vi "AG33XXX.enable output.vi"(0 "i ref in":refnum<vi>, 2 "outputEnable":bool, 3 "ms timeout (10000)":i32=10000, 5 "error in (no error)":errorcluster) -> (14 "i ref out":refnum<vi>, 17 "timed out":bool, 19 "error out":errorcluster)   [LabVIEW 2014, in "AG33XXX.lvlib"]
doc: "Enables the output of the device."
uses:
  AG33XXX.lvlib
  CS_Core/CSApplicationBaseClasses/AFGBase/AFGBase.serviceType.ctl
  CS_Core/CSApplicationBaseClasses/AFGBase/AFGBase.directionType.ctl
  CSlibraries/UtilityLib/UtilityLib.valueStatus.ctl
  CS_Core/CSApplicationBaseClasses/DeviceBase/DeviceBase.lvlib
  CS_Core/CSApplicationBaseClasses/AFGBase/AFGBase.lvlib
  CSlibraries/UtilityLib/UtilityLib.lvlib
  instr.lib/agilent_33xxx_series/Agilent 33XXX Series/Agilent 33XXX Series.lvlib
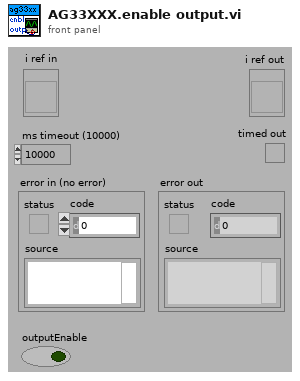
[diagram p1: front panel]
types:
  T1 = typedef "UtilityLib.lvlib/UtilityLib.valueStatus.ctl" = enum16{"no info available", "stand by/off", "on", "warning", "alarm/malfunction", "not implemented", "user action required", "important information", "system default", "control default", "indicator default", "button default"}
  T2 = typedef "AFGBase.lvlib/AFGBase.directionType.ctl" = enum16{"unknown", "update actual value", "update nominal value", "update both"}
  T3 = typedef "AFGBase.lvlib/AFGBase.serviceType.ctl" = enum16{"frequency", "amplitude", "phase", "DCOffset", "enableOutput", "trigger", "waveformType"}
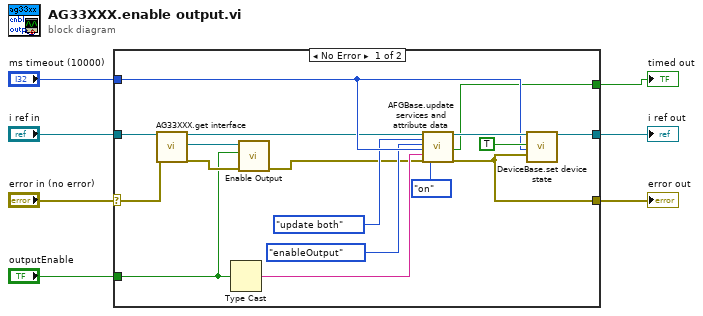
[diagram p0: block diagram]
diagram:
  n1 = case shown="No Error" "error in (no error)" {
    selector: "error in (no error)" -> [w14 w25]
    tunnel: [w24 w26] -> w7
    tunnel: "ms timeout (10000)" -> [w20 _]
    tunnel: "i ref in" -> [w15 w26]
    tunnel: [w21 w25] -> w3
    tunnel: "outputEnable" -> [w10 _]
    tunnel: [w8 _] -> w1
    frame No Error {
      n2 = call "AG33XXX.get interface.vi"("i ref in"=w15, "error in (no error)"=w14) -> ("i ref out"=w13:refnum<vi>, "interface"=w11:refnum<visa-resource-name>, "error out"=w12:errorcluster)  [unwired: 15 in]
      n3 = Type Cast(x=w10) -> (*(type *) &x=w18:string)  [unwired: 1 in]
      n4 = call "Enable Output.vi"("error in (no error)"=w12, "Enable Output (T: Enable)"=w10, "VISA resource name"=w11) -> ("error out"=w9:errorcluster)  [unwired: 7 in, 1 out]
      n5 = call "AFGBase.update services and attribute data.vi"("i ref in"=w13, "direction"=AFGBase.directionType."update both", "service"=AFGBase.serviceType."enableOutput", "ms timeout (10000)"=w20, "value"=w18, "error in (no error)"=w9, "quality"=UtilityLib.valueStatus."on") -> ("i ref out"=w22:refnum<vi>, "timed out"=w8:bool, "error out"=w21:errorcluster)  [unwired: 10 in]
      n6 = call "DeviceBase.set device state.vi"("i ref in"=w22, "implicit"=TRUE, "ms timeout (10000)"=w20, "device error"=w21) -> ("i ref out"=w24:refnum<vi>)  [unwired: 13 in, 2 out]
    }
    frame Error {
    }
  }
  "error out" <- w3
  "i ref out" <- w7
  "timed out" <- w1
